vi "Realtime Clock-Direct.vi"() -> ()   [LabVIEW 2009]
uses:
  <vilib>/NXT/Block Support/NXT_InputPort.ctl
  <vilib>/NXT/Subs/LVHSConnector.ctl
panel:
  out "Status":bool caption="Success?"
  out "NXT dup":T1 caption="NXT"
  in  "NXT":T1
  in  "stop":bool
  out "Month":dbl
  out "Minute":dbl
  out "Year":dbl
  out "Hour":dbl
  out "Date":dbl
  out "Second":dbl
  out "date string":string
  out "time string":string
  in  "Input Port":T2 items=["Port 1", "Port 2", "Port 3", "Port 4"]
  # "mindsensors.com\nCopyright (c) 2009 by mindsensors.com\nEmail: info (<at>) mindsensors (<dot>) com\n\nThis program is free software. You can redistribute it and/or modify\nit under the terms of the GNU General Public License as published by\nthe Free Software Foundation; version 3 of the License.\nRead the license at: http://www.gnu.org/licenses/gpl.txt"
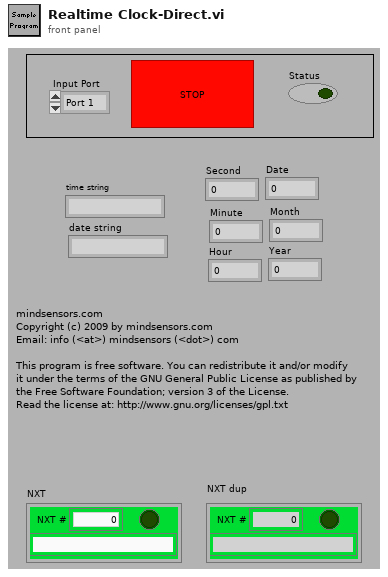
[diagram p1: front panel]
types:
  T1 = typedef "LVHSConnector.ctl" = cluster{"error":errorcluster, "address":string, "NXT #":i32, "Show Error":bool}
  T2 = typedef "NXT_InputPort.ctl" = u8
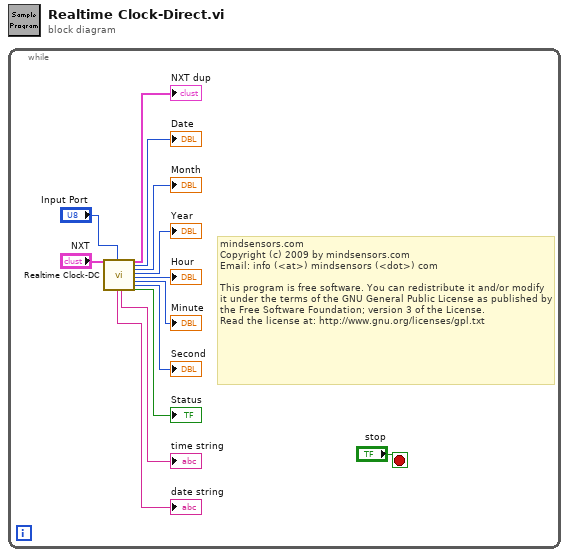
[diagram p0: block diagram]
diagram:
  n1 = while {
    stop <- "stop" stop-if-true
    # "mindsensors.com\nCopyright (c) 2009 by mindsensors.com\nEmail: info (<at>) mindsensors (<dot>) com\n\nThis program is free software. You can redistribute it and/or modify\nit under the terms of the GNU General Public License as published by\nthe Free Software Foundation; version 3 of the License.\nRead the license at: http://www.gnu.org/licenses/gpl.txt"
    n2 = call "Realtime Clock-DC.vi"("NXT"="NXT", "Input Port"="Input Port") -> ("date string"=→"date string":string, "time string"=→"time string":string, "NXT dup"=→"NXT dup":T1, "date"=→"Date":i8, "month"=→"Month":i8, "Year"=→"Year":i16, "Hour"=→"Hour":i8, "minute"=→"Minute":i8, "second"=→"Second":i8, "Status"=→"Status":bool)  [unwired: 16 in]
  }
